vi "Write to file (CLTC-76ZM0M1's conflicted copy 2014-09-09).vi"(8 "error in (no error)":errorcluster, 9 "Data Cluster":T4, 10 "Test Case":T5, 11 "Don't wait for stabilizatoin":bool) -> (0 "error out":errorcluster)   [LabVIEW 2013]
uses:
  Test Case.ctl
  Power Values.ctl
  <vilib>/addons/Electrical Power/Basic/Measurement/subVIs/basic_Power Value.ctl
  Stabilization.ctl
  <vilib>/addons/Electrical Power/Basic/NI_EP_Basic.lvlib
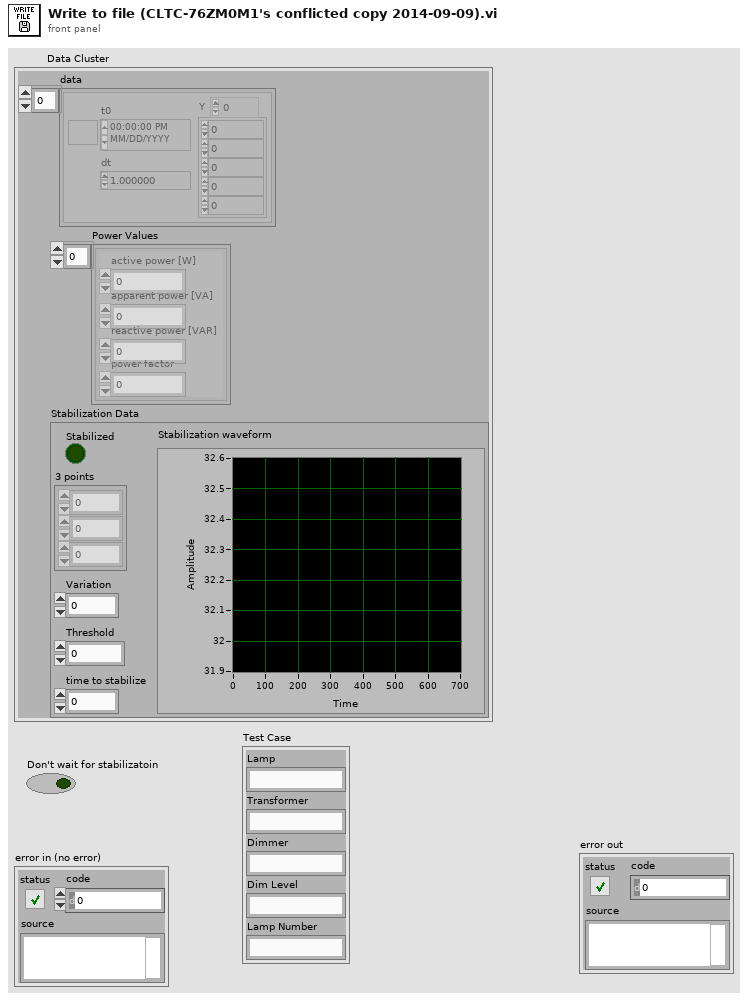
[diagram p1: front panel]
types:
  T1 = typedef "Power Values.ctl" = T2[]
  T2 = typedef "NI_EP_Basic.lvlib/basic_Power Value.ctl" = cluster{"active power [W]":dbl, "apparent power [VA]":dbl, "reactive power [VAR]":dbl, "power factor":dbl}
  T3 = typedef "Stabilization.ctl" = cluster{"Stabilization waveform":waveform(dbl), "Variation":dbl, "Stabilized":bool, "Threshold":dbl, "time to stabilize":dbl, "3 points":dbl[]}
  T4 = cluster{"data":waveform(dbl)[], "Power Values":T1, "Stabilization Data":T3}
  T5 = typedef "Test Case.ctl" = cluster{"Lamp":string, "Transformer":string, "Dimmer":string, "Dim Level":string, "Lamp Number":string}
  T6 = enum16{"open", "open or create", "create or replace", "create", "open (read-only)"}
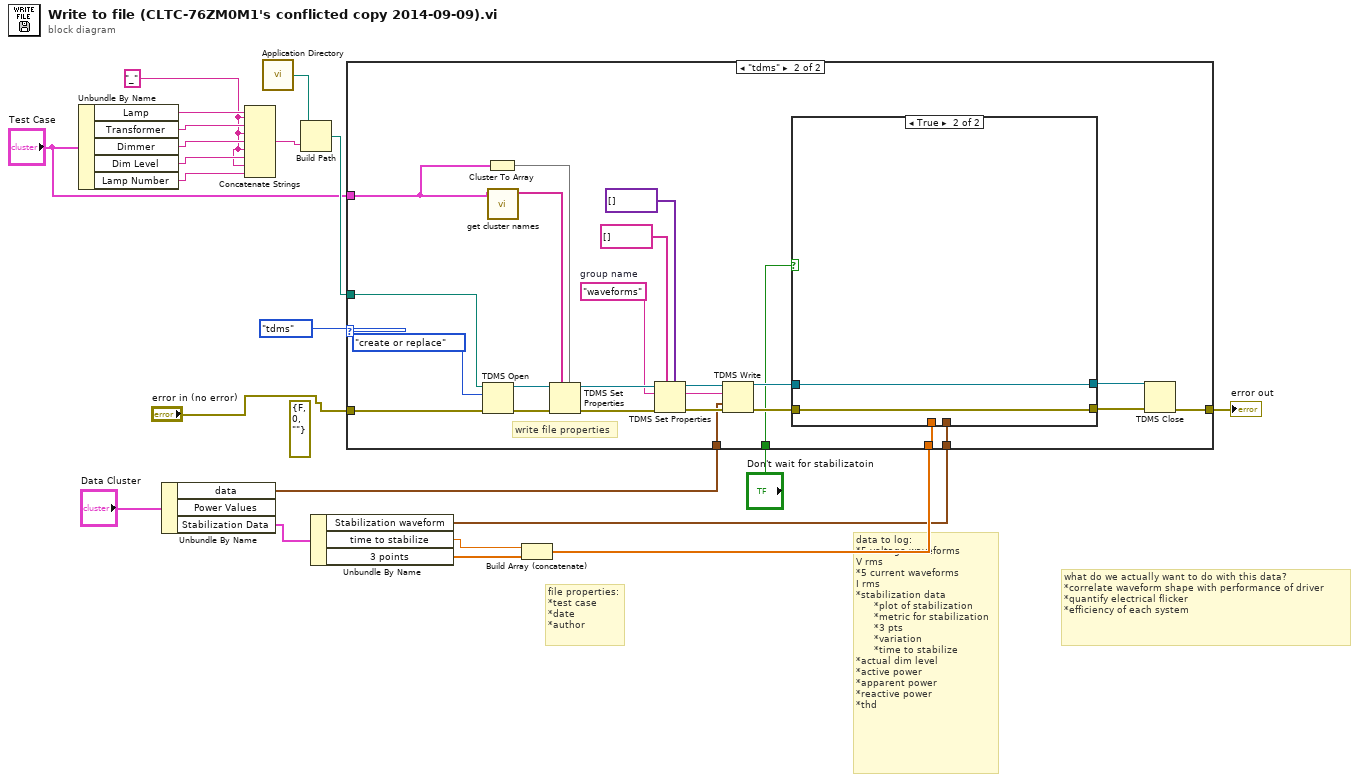
[diagram p0: block diagram]
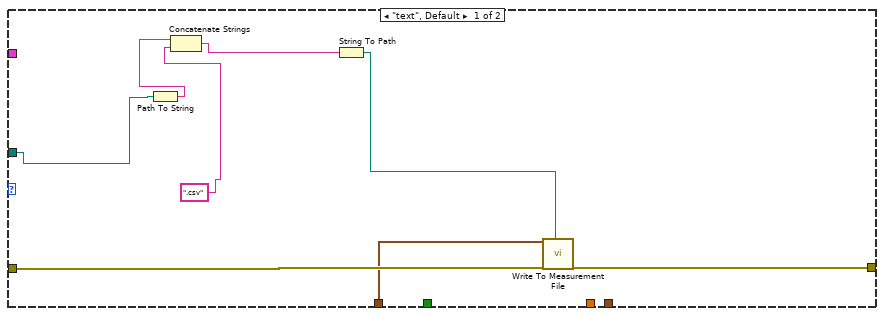
[diagram p2: hidden frame]
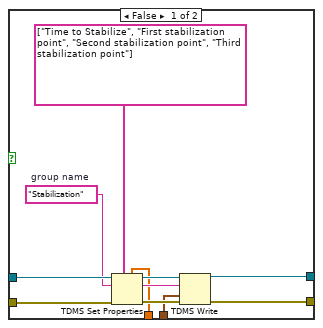
[diagram p3: hidden frame]
diagram:
  (unwired) errorcluster {"status"=FALSE, "code"=0, "source"=""} ("error in (no error)")
  w17 = "_"
  # "what do we actually want to do with this data?\n*correlate waveform shape with performance of driver\n*quantify electrical flicker\n*efficiency of each system"
  # "data to log:\n*5 voltage waveforms\nV rms\n*5 current waveforms\nI rms\n*stabilization data\n      *plot of stabilization\n      *metric for stabilization\n      *3 pts\n      *variation\n      *time to stabilize\n*actual dim level\n*active power\n*apparent power\n*reactive power\n*thd"
  # "file properties:\n*test case\n*date\n*author"
  n1 = Unbundle By Name("Test Case") -> ("Lamp"=w21:string, "Transformer"=w20:string, "Dimmer"=w19:string, "Dim Level"=w18:string, "Lamp Number"=w16:string)
  n2 = Unbundle By Name("Data Cluster") -> ("data"=w8:waveform(dbl)[], "Stabilization Data"=w7:T3)  [unwired: 1 out]
  n3 = Concatenate Strings(w21, w17, w20, w17, w19, w17, w18, w17, w16) -> (w14:string)
  n4 = call <vilib>:"Application Directory.vi"() -> ("Application Directory"=w15:path)
  n5 = Build Path(base path=w15, name or relative path=w14) -> (appended path=w13:path)
  n6 = Unbundle By Name(w7) -> ("Stabilization waveform"=w3:waveform(dbl), "time to stabilize"=w6:dbl, "3 points"=w5:dbl[])
  n7 = Build Array (concatenate)(w6, w5) -> (w4:dbl[])
  n8 = case shown="\"tdms\"" enum16{"tdms", "text"}."tdms" {
    tunnel: w13 -> [w26 w50]
    tunnel: "error in (no error)" -> [w29 w51]
    tunnel: [w28 w49] -> w11
    tunnel: w8 -> [w27 w39]
    tunnel: "Test Case" -> [_ w46]
    tunnel: w4 -> [_ w36]
    tunnel: w3 -> [_ w35]
    tunnel: "Don't wait for stabilizatoin" -> [_ w32]
    frame "text", Default {
      n9 = Path To String(path=w26) -> (string=w25:string)
      n10 = Concatenate Strings(w25, ".csv") -> (w23:string)
      n11 = String To Path(string=w23) -> (path=w22:path)
      n12 = call "Write To Measurement File"("Signals"=w27, "error in (no error)"=w29, "Filename"=w22) -> ("error out"=w28:errorcluster)  [unwired: 14 in, 2 out]
    }
    frame "tdms" {
      w43 = "waveforms"  # group name
      # "write file properties"
      n13 = TDMS Open(8:w51, 10:T6."create or replace" ("operation (0:open)"), 11:w50) -> (0:w54:errorcluster, 3:w52:refnum<k34>)  [unwired: 4 in]
      n14 = Cluster To Array(cluster=w46) -> (array=w48:string[])
      n15 = call "get cluster names.vi"("Variant"=w46) -> ("Data Labels Array"=w47:string[])  [unwired: 10 in]
      n16 = TDMS Set Properties(5:w48, 7:w47, 8:w54, 11:w52) -> (0:w44:errorcluster, 3:w45:refnum<k34>)  [unwired: 2 in, 2 out]
      n17 = TDMS Set Properties(5:variant[] [] ("property values"), 7:string[] [] ("property names"), 8:w44, 10:w43, 11:w45) -> (0:w41:errorcluster, 2:w40:string, 3:w42:refnum<k34>)  [unwired: 1 in, 1 out]
      n18 = TDMS Write(0:w42, 5:w40, 9:w39, 11:w41) -> (4:w37:refnum<k34>, 15:w38:errorcluster)  [unwired: 2 in, 2 out]
      n19 = case shown="True" w32 {
        tunnel: w38 -> [w62 w66]
        tunnel: w37 -> [w61 w67]
        tunnel: w36 -> [w59 _]
        tunnel: w35 -> [w57 _]
        tunnel: [w56 w67] -> w34
        tunnel: [w55 w66] -> w33
        frame False {
          w60 = "Stabilization"  # group name
          n20 = TDMS Set Properties(5:w59, 7:string[] ["Time to Stabilize", "First stabilization point", "Second stabilization point", "Third stabilization point"] ("property names"), 8:w62, 10:w60, 11:w61) -> (0:w64:errorcluster, 2:w65:string, 3:w63:refnum<k34>)  [unwired: 1 in, 1 out]
          n21 = TDMS Write(0:w63, 5:w65, 9:w57, 11:w64) -> (4:w56:refnum<k34>, 15:w55:errorcluster)  [unwired: 2 in, 2 out]
        }
        frame True {
        }
      }
      n22 = TDMS Close(8:w33, 11:w34) -> (0:w49:errorcluster)  [unwired: 1 out]
    }
  }
  "error out" <- w11
